vi "Get Value and Limit Display From Measure Results.vi"(1 "Measure Results":T2[](array[typedef])) -> (0 "Value Limit Data":T1)   [LabVIEW 2015, in "Execution.lvclass"]
uses:
  Execution.lvclass
  STEP_MEASURE_RESULT.ctl
  Step/OUTPUT_DATA_TYPE.ctl
  OutputUI/OUTPUT_CHECK_TYPE.ctl
  Step/STEP_STATUS.ctl
  Step.lvclass
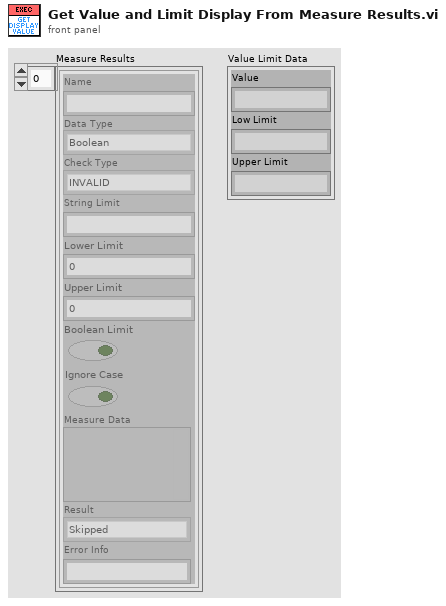
[diagram p1: front panel]
types:
  T1 = cluster{"Value":string, "Low Limit":string, "Upper Limit":string}
  T2 = typedef "Execution.lvclass/STEP_MEASURE_RESULT.ctl" = cluster{"Name":string, "Data Type":T3, "Check Type":T4, "String Limit":string, "Lower Limit":dbl, "Upper Limit":dbl, "Boolean Limit":bool, "Ignore Case":bool, "Measure Data":variant, "Result":T5, "Error Info":string}
  T3 = typedef "Step.lvclass/OUTPUT_DATA_TYPE.ctl" = enum16{"Boolean", "String", "Numeric", "Other"}
  T4 = typedef "Step.lvclass/OUTPUT_CHECK_TYPE.ctl" = enum16{"INVALID", "DO_NOT_CHECK", "RECORD", "VARIABLE", "EQUAL", "NOT_EQUAL", "STR_CONTAINS", "STR_START_WITH", "STR_END_WITH", "STR_REGEX_MATCH", "NUM_GT", "NUM_LT", "NUM_GE", "NUM_LE", "NUM_RANGE", "NUM_RANGE_BDY"}
  T5 = typedef "Step.lvclass/STEP_STATUS.ctl" = enum16{"Skipped", "Done", "Passed", "Failed", "Error"}
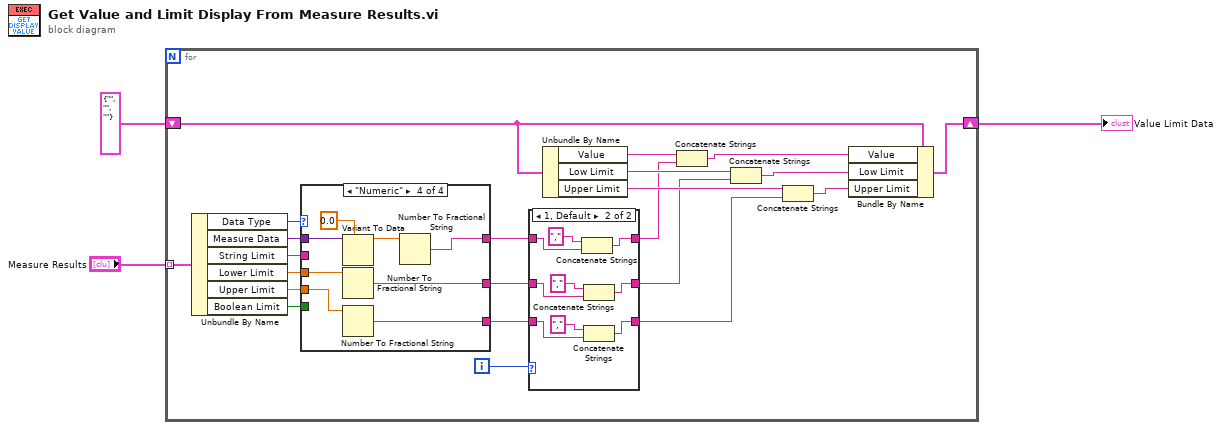
[diagram p0: block diagram]
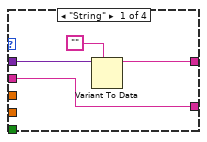
[diagram p3: hidden frame]
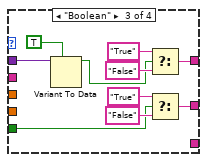
[diagram p5: hidden frame]
diagram:
  n1 = for {
    tunnel: "Measure Results" -> [w25] mode=indexing
    shift-right: [w16] -> w1
    shift-left: T1 {"Value"="", "Low Limit"="", "Upper Limit"=""} ("Value Limit Data") -> [w15]
    i -> [w10]
    n2 = Unbundle By Name(w25) -> ("Data Type"=w24:T3, "Measure Data"=w23:variant, "String Limit"=w22:string, "Lower Limit"=w21:dbl, "Upper Limit"=w20:dbl, "Boolean Limit"=w19:bool)
    n3 = case shown="\"Numeric\"" w24 {
      tunnel: w23 -> [w41 _ w51 w59]
      tunnel: [w39 _ w42 w52] -> w9
      tunnel: w22 -> [w38 _ _ _]
      tunnel: w21 -> [_ _ _ w57]
      tunnel: w20 -> [_ _ _ w55]
      tunnel: w19 -> [_ _ w44 _]
      tunnel: [w38 _ w43 w56] -> w7
      tunnel: [_ _ _ w54] -> w5
      frame "String" {
        n4 = Variant To Data(type="", Variant=w41) -> (data=w39:string)  [unwired: 1 in, 1 out]
      }
      frame "Other" {
      }
      frame "Boolean" {
        n5 = Variant To Data(type=TRUE, Variant=w51) -> (data=w47:bool)  [unwired: 1 in, 1 out]
        n6 = Select(t="True", s=w47, f="False") -> (s? t:f=w42:string)
        n7 = Select(t="True", s=w44, f="False") -> (s? t:f=w43:string)
      }
      frame "Numeric" {
        n8 = Variant To Data(type=0.0, Variant=w59) -> (data=w53:dbl)  [unwired: 1 in, 1 out]
        n9 = Number To Fractional String(number=w57) -> (F-format string=w56:string)  [unwired: 3 in]
        n10 = Number To Fractional String(number=w55) -> (F-format string=w54:string)  [unwired: 3 in]
        n11 = Number To Fractional String(number=w53) -> (F-format string=w52:string)  [unwired: 3 in]
      }
    }
    n12 = case shown="1, Default" w10 {
      tunnel: w9 -> [w28 w36]
      tunnel: [w28 w35] -> w8
      tunnel: [w27 w33] -> w6
      tunnel: w7 -> [w27 w32]
      tunnel: w5 -> [w26 w29]
      tunnel: [w26 w30] -> w4
      frame 0 {
      }
      frame 1, Default {
        n13 = Concatenate Strings(",", w36) -> (w35:string)
        n14 = Concatenate Strings(",", w32) -> (w33:string)
        n15 = Concatenate Strings(",", w29) -> (w30:string)
      }
    }
    n16 = Unbundle By Name(w15) -> ("Value"=w18:string, "Low Limit"=w14:string, "Upper Limit"=w12:string)
    n17 = Concatenate Strings(w18, w8) -> (w17:string)
    n18 = Concatenate Strings(w14, w6) -> (w13:string)
    n19 = Concatenate Strings(w12, w4) -> (w11:string)
    n20 = Bundle By Name(cluster=w15, "Value"=w17, "Low Limit"=w13, "Upper Limit"=w11) -> (w16:T1)
  }
  "Value Limit Data" <- w1
